vi "ZCAN_ClearBuffer.vi"(8 "error in (no error)":errorcluster caption="错误输入（无错误）", 10 "can_index_handle":u32) -> (0 "error out":errorcluster caption="错误输出", 2 "ClearBuffer_success?":bool)   [LabVIEW 2011, in "zlgcan.lvlib"]
doc: "该函数用于清除库接收缓冲区。"
uses:
  zlgcan.lvlib
  bin/ControlCANFD.dll
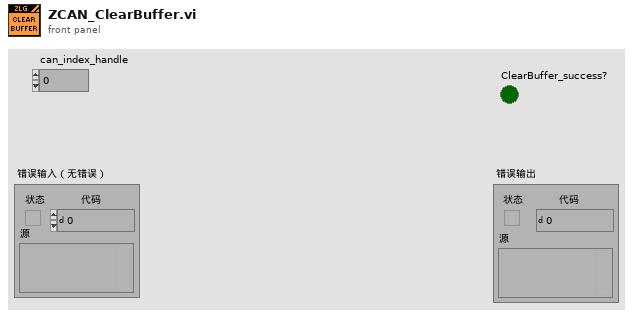
[diagram p1: front panel]
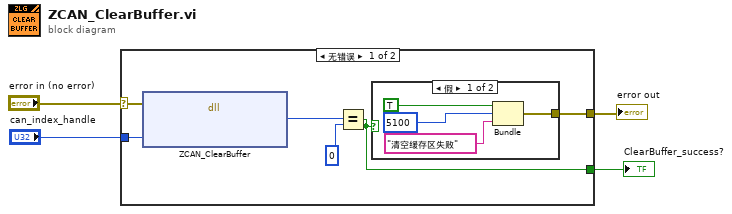
[diagram p0: block diagram]
diagram:
  n1 = case shown="无错误" "error in (no error)" {
    selector: "error in (no error)" -> [w5 w15]
    tunnel: [w8 w15] -> w3
    tunnel: "can_index_handle" -> [w10 _]
    tunnel: [w6 _] -> w1
    frame No Error {
      n2 = dll-call lib="C:/Users/ttc52/Desktop/DHC FD LV2018/LABIVIEW2011 CANFD Tool_V1.2.4_x86_20250428/bin/ControlCANFD.dll" fn="ZCAN_ClearBuffer" ("ZCAN_StartCAN")(error in=w5, "can_handle"=w10) -> ("return"=w7:u32)  [unwired: 3 in, 2 out]
      n3 = Equal?(x=w7, y=0) -> (x = y?=w6:bool)
      n4 = case shown="假" w6 {
        tunnel: [w11 _] -> w8
        frame False {
          n5 = Bundle("status"=TRUE, "code"=5100, "消息"="清空缓存区失败") -> (w11:cluster{"status":bool, "code":i32, "消息":string})  [unwired: 1 in]
        }
        frame True {
        }
      }
    }
    frame Error {
    }
  }
  "error out" <- w3
  "ClearBuffer_success?" <- w1
